vi "Open.vi"(8 "error in (no error)":errorcluster, 11 "MelsecTCP in":refnum<class "InovanceModbusTcp.lvclass">) -> (0 "error out":errorcluster, 3 "MelsecTCP out":refnum<class "InovanceModbusTcp.lvclass">)   [LabVIEW 2020, in "HslCommunication.lvlib" / "InovanceModbusTcp.lvclass"]
uses:
  InovanceModbusTcp.lvclass
  InovanceModbusTcp.lvclass/InovanceModbusTcp.ctl
  E:/Git/Libraries/develop/HslCommunication/_Dependenciecs/HslCommunication.dll
  _Dependenciecs/HslCommunication.dll
  Read series.vi
  Read ipAddress.vi
  Read port.vi
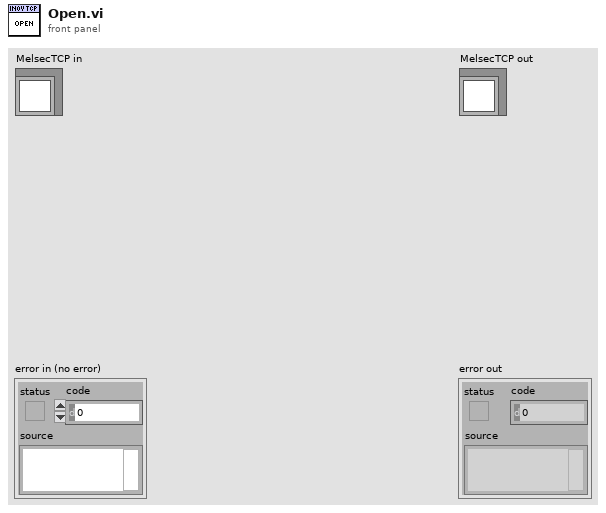
[diagram p1: front panel]
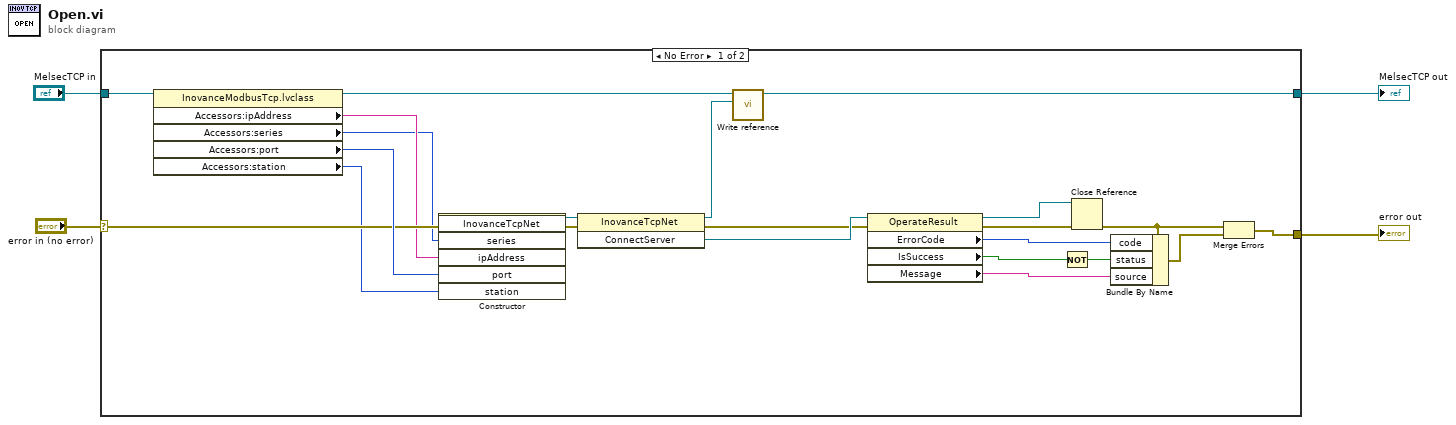
[diagram p0: block diagram]
diagram:
  n1 = case shown="No Error" "error in (no error)" {
    selector: "error in (no error)" -> [w10 w28]
    tunnel: "MelsecTCP in" -> [w26 w27]
    tunnel: [w6 w27] -> w1
    tunnel: [w20 w28] -> w2
    frame No Error {
      n2 = property class="InovanceModbusTcp.lvclass"(reference=w26) -> (reference out=w12:refnum<class "InovanceModbusTcp.lvclass">, "Accessors:ipAddress"=w9:string, "Accessors:series"=w7:i32, "Accessors:port"=w11:i32, "Accessors:station"=w8:u8)  [unwired: 1 in, 1 out]
      n3 = constructor class="InovanceTcpNet"(error in=w10, "series"=w7, "ipAddress"=w9, "port"=w11, "station"=w8) -> (reference out=w15:refnum<k24>, error out=w14:errorcluster)  [unwired: 2 in, 5 out]
      n4 = invoke class="InovanceTcpNet" method="ConnectServer"(reference=w15, error in=w14) -> (reference out=w5:refnum<k24>, error out=w17:errorcluster, "ConnectServer"=w19:refnum<k24>)  [unwired: 1 in]
      n5 = call-dynamic "Write reference.vi"("reference"=w5, "MelsecTCP in"=w12) -> ("MelsecTCP out"=w6:refnum<class "InovanceModbusTcp.lvclass">)  [unwired: 8 in, 1 out]
      n6 = property class="OperateResult"(reference=w19, error in=w17) -> (reference out=w18:refnum<k24>, error out=w16:errorcluster, "ErrorCode"=w23:i32, "IsSuccess"=w13:bool, "Message"=w21:string)
      n7 = Not(x=w13) -> (.not. x?=w22:bool)
      n8 = Close Reference(reference=w18, error in (no error)=w16) -> (error out=w24:errorcluster)
      n9 = Bundle By Name(cluster=w24, "code"=w23, "status"=w22, "source"=w21) -> (w25:errorcluster)
      n10 = Merge Errors(w24, w25) -> (w20:errorcluster)
    }
    frame Error {
    }
  }
  "error out" <- w2
  "MelsecTCP out" <- w1
